vi "processData.vi"(8 "error in (no error)":errorcluster, 10 "model":refnum<class "Model.lvclass">, 11 "MovingToNewForceState in":refnum<class "MovingToNewForceState.lvclass">) -> (0 "error out":errorcluster, 2 "model 2":refnum<class "Model.lvclass">, 3 "MovingToNewForceState out":refnum<class "MovingToNewForceState.lvclass">)   [LabVIEW 2013, in "MovingToNewForceState.lvclass"]
uses:
  MovingToNewForceState.lvclass
  Model/Model/Model.lvclass
  ExecutingCycleState/ExecutingCycleState.lvclass
  Typedefs/StateSelector.ctl
  Typedefs/M2AADTTypedefs.lvlib
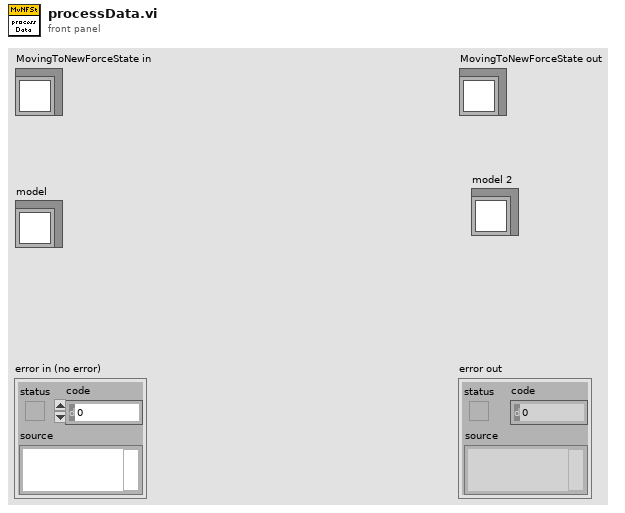
[diagram p1: front panel]
types:
  T1 = typedef "M2AADTTypedefs.lvlib/StateSelector.ctl" = enum16{"EndingCycleState", "FaultState", "InteractiveMotionState", "MovingToNewForceState", "OffState", "PausingState", "StandbyState", "StoppedState"}
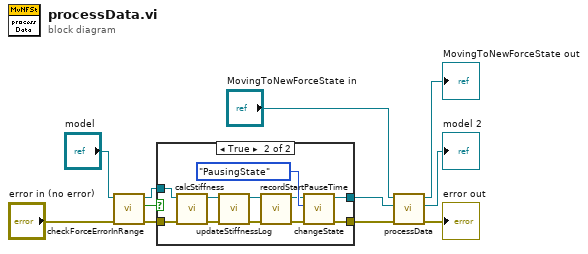
[diagram p0: block diagram]
diagram:
  n1 = call "checkForceErrorInRange.vi"("error in (no error)"="error in (no error)", "Model in"="model") -> ("error out"=w3:errorcluster, "inRangeIsTrue"=w4:bool, "Model out"=w5:refnum<class "Model.lvclass">)  [unwired: 7 in]
  n2 = case shown="True" w4 {
    tunnel: w5 -> [w13 w19]
    tunnel: w3 -> [w12 w18]
    tunnel: [w12 w24] -> w2
    tunnel: [w13 w23] -> w1
    frame False {
    }
    frame True {
      n3 = call "calcStiffness.vi"("error in (no error)"=w18, "Model in"=w19) -> ("error out"=w15:errorcluster, "Model out"=w17:refnum<class "Model.lvclass">)  [unwired: 8 in]
      n4 = call "updateStiffnessLog.vi"("error in (no error)"=w15, "Model in"=w17) -> ("error out"=w14:errorcluster, "Model out"=w16:refnum<class "Model.lvclass">)  [unwired: 8 in]
      n5 = call "recordStartPauseTime.vi"("error in (no error)"=w14, "Model in"=w16) -> ("error out"=w20:errorcluster, "Model out"=w21:refnum<class "Model.lvclass">)  [unwired: 8 in]
      n6 = call "changeState.vi"("error in (no error)"=w20, "State:"=StateSelector."PausingState", "Model in"=w21) -> ("error out"=w24:errorcluster, "Model out"=w23:refnum<class "Model.lvclass">)  [unwired: 7 in]
    }
  }
  n7 = call-parent "processData.vi"("error in (no error)"=w2, "model"=w1, "ControlledMotionState in"="MovingToNewForceState in") -> ("error out"=→"error out":errorcluster, "model 2"=→"model 2":refnum<class "Model.lvclass">, "ControlledMotionState out"=→"MovingToNewForceState out":refnum<class "MovingToNewForceState.lvclass">)  [unwired: 6 in]
